vi "SDCP SMF Receiver and Transmitter - Tx Table Elements FGV.vi"(3 "error in (no error)":errorcluster, 4 "Command":enum16{"Read", "Write"}(ring), 5 "Table elements in":T1[](array[typedef])) -> (0 "error out":errorcluster, 2 "Table elements out":T1[](array[typedef]))   [LabVIEW 2020]
uses:
  Typedefs/SDCP SMF Receiver and Transmitter - Transmit Table Element.ctl
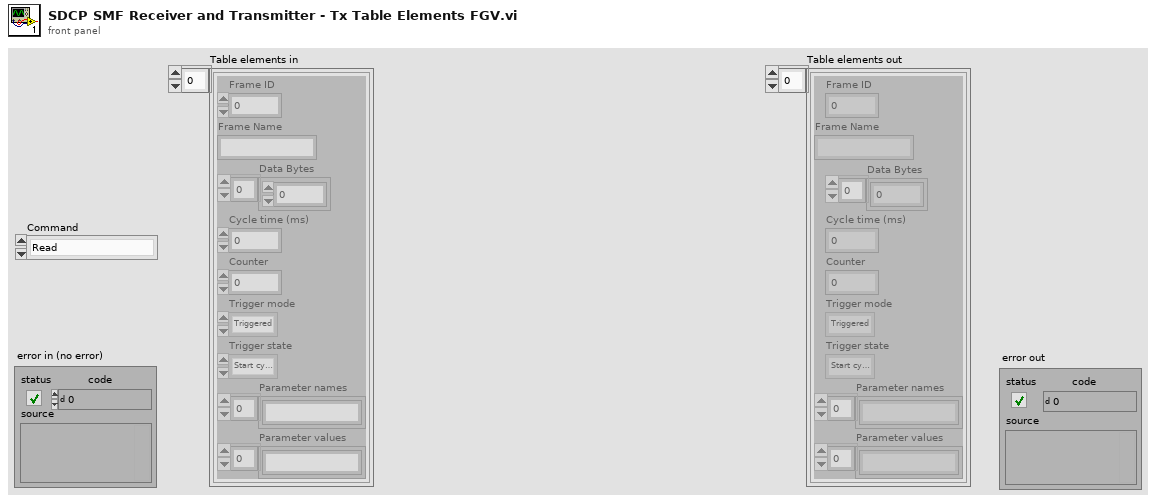
[diagram p1: front panel]
types:
  T1 = typedef "SDCP SMF Receiver and Transmitter - Transmit Table Element.ctl" = cluster{"Frame ID":i32, "Frame Name":string, "Data Bytes":u8[], "Cycle time (ms)":i32, "Counter":i32, "Trigger mode":enum16{"Triggered", "Cyclic"}, "Trigger state":enum16{"Stop cyclic trigger", "Start cyclic trigger", "Stop single trigger", "Start single trigger"}, "Parameter names":string[], "Parameter values":string[]}
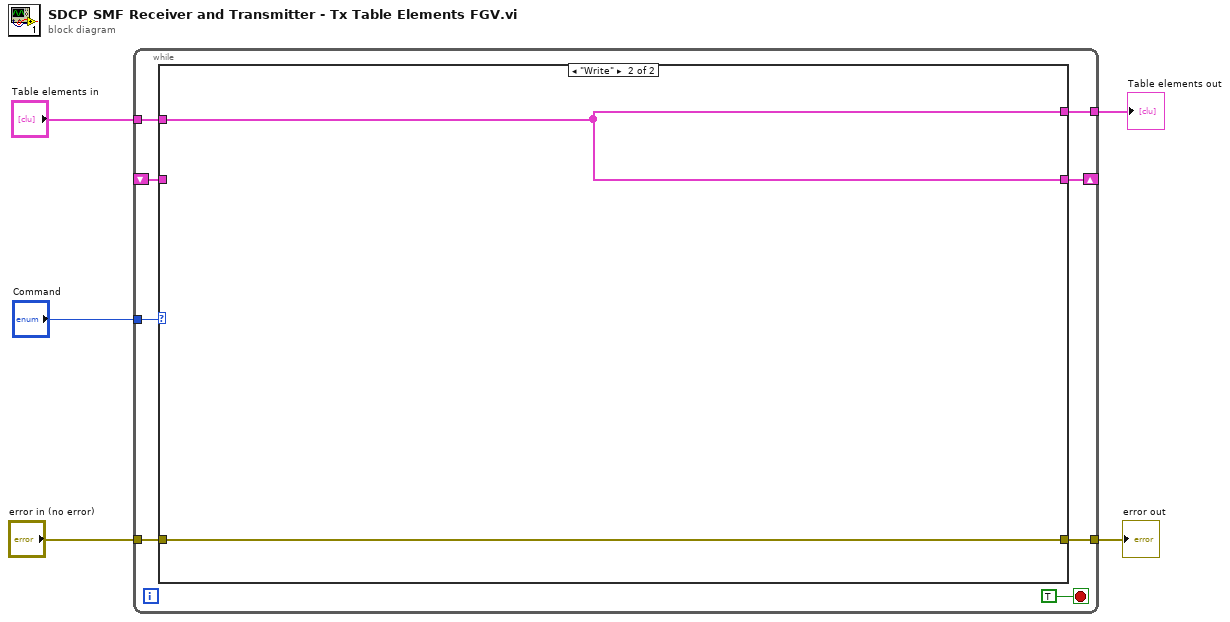
[diagram p0: block diagram]
diagram:
  n1 = while {
    tunnel: "error in (no error)" -> [w8]
    tunnel: "Table elements in" -> [w11]
    tunnel: "Command" -> [w13]
    shift-right: [w12] -> _
    shift-left: _ -> [w10]
    tunnel: [w9] -> w2
    tunnel: [w7] -> w1
    stop <- TRUE stop-if-true
    n2 = case shown="\"Write\"" w13 {
      tunnel: [w15 w17] -> w12
      tunnel: w11 -> [_ w17]
      tunnel: w10 -> [w15 _]
      tunnel: [w15 w17] -> w9
      tunnel: w8 -> [w14 w16]
      tunnel: [w14 w16] -> w7
      frame "Read", Default {
      }
      frame "Write" {
      }
    }
  }
  "error out" <- w1
  "Table elements out" <- w2
